vi "week02_Ex02.vi"() -> ()   [LabVIEW 2017]
panel:
  out "Errer":bool
  out "End":bool
  out "X-Y":i16
  out "Counter":i16
  in  "Boolean":bool
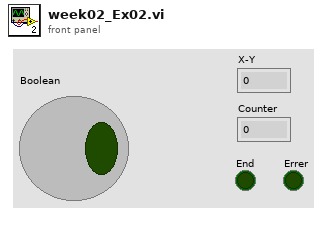
[diagram p1: front panel]
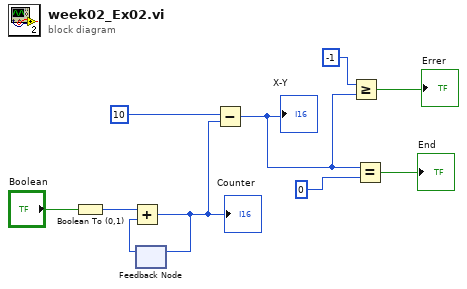
[diagram p0: block diagram]
diagram:
  n1 = Boolean To (0,1)(Boolean="Boolean") -> (0, 1=w9:i16)
  n2 = feedback #1() -> (w8:i16)  [unwired: 1 in]
  n3 = Add(x=w9, y=w8) -> (x+y=w7:i16)
  "Counter" <- w7
  n4 = feedback-in #1(w7) -> ()
  n5 = Subtract(x=10, y=w7) -> (x-y=w3:i32)
  "X-Y" <- w3
  n6 = Greater Or Equal?(x=-1, y=w3) -> (x >= y?=→"Errer":bool)
  n7 = Equal?(x=w3, y=0) -> (x = y?=→"End":bool)
